vi "Cron Next (Quartz-compatible).vi"(9 "Nb Occurences (min: 1)":u16=1 min=1, 10 "Reference timestamp (Now)":timestamp, 11 "Cron Expression":string="* * * * ? *") -> (1 "Occurences":timestamp[](array[timestamp]), 2 "Next Occurence":timestamp, 3 "syntax valid?":bool)   [LabVIEW 2013, in "openCron.lvlib"]
uses:
  openCron.lvlib
  Cron.Quartz/Cron.Quartz.lvclass
  Cron/Cron.lvclass
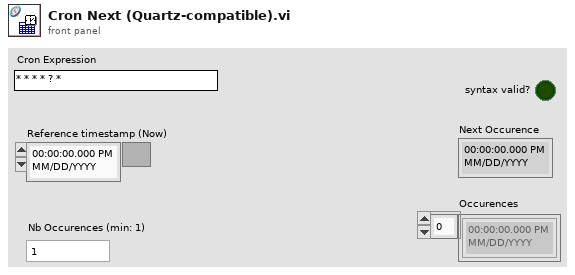
[diagram p1: front panel]
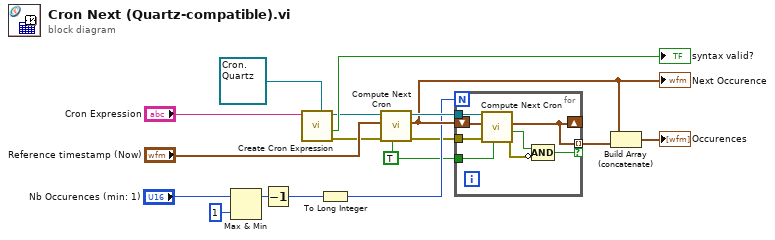
[diagram p0: block diagram]
diagram:
  w3 = TRUE ("Ignore DST?")
  n1 = Max & Min(x="Nb Occurences (min: 1)", y=u16 1) -> (max(x,y)=w9:u16)  [unwired: 1 out]
  n2 = Decrement(x=w9) -> (x-1=w8:u16)
  n3 = call "Create Cron Expression.vi"("Cron in"=refnum<class "Cron.Quartz.lvclass"> refnum ("openCron.lvlib:Cron.Quartz.lvclass"), "Cron Expression"="Cron Expression") -> ("error out"=w2:errorcluster, "expression valid"=→"syntax valid?":bool, "Cron out"=w14:refnum<class "Cron.Quartz.lvclass">)  [unwired: 7 in]
  n4 = To Long Integer(number=w8) -> (32bit integer=w4:i32)
  n5 = call "Compute Next Cron.vi"("Ignore DST?"=w3, "error in (no error)"=w2, "Time Stamp (Now)"="Reference timestamp (Now)", "Cron in"=w14) -> ("error out"=w1:errorcluster, "Next Occurence"=w6:timestamp, "Cron out"=w12:refnum<class "Cron.Quartz.lvclass">)  [unwired: 4 in, 1 out]
  "Next Occurence" <- w6
  n6 = for {
    N: w4 -> [_]
    shift-right: [w23] -> _
    shift-left: w6 -> [w25]
    tunnel: w12 -> [w24]
    tunnel: [w23] -> w7 mode=indexing if=w18
    tunnel: w3 -> [w22]
    tunnel: w1 -> [w21]
    n7 = call "Compute Next Cron.vi"("Ignore DST?"=w22, "error in (no error)"=w21, "Time Stamp (Now)"=w25, "Cron in"=w24) -> ("error out"=w20:errorcluster, "Occurence found"=w19:bool, "Next Occurence"=w23:timestamp)  [unwired: 4 in, 1 out]
    n8 = Compound Arithmetic op=AND(w19, invert w20) -> (w18:bool)
  }
  n9 = Build Array (concatenate)(w6, w7) -> (→"Occurences":timestamp[])
